vi "Starting.vi"(4 "Queue of Error":refnum<queue>, 6 "Queue of Self Attributes":refnum<queue>, 7 "Actor in":refnum<class "Actor.lvclass">, 10 "Attributes":refnum<class "Attributes.lvclass">) -> (0 "Error out":errorcluster, 5 "Actor out":refnum<class "Actor.lvclass">)   [LabVIEW 2025, in "jettl.lvlib" / "Transport.lvlib" / "Event.lvlib"]
uses:
  Event.lvlib
  Actor/Actor.lvclass
  Attributes/Attributes/Attributes.lvclass
  jettl.lvlib
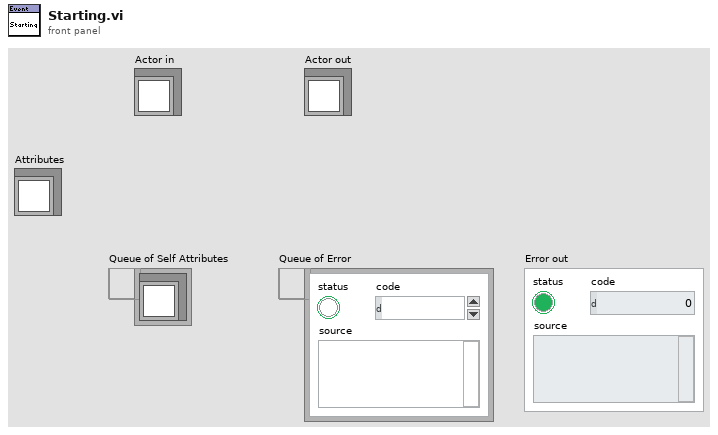
[diagram p1: front panel]
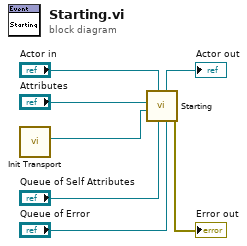
[diagram p0: block diagram]
diagram:
  n1 = call "Init Transport.vi"() -> ("Transport"=w1:refnum<class "Transport.lvclass">)  [unwired: 11 in]
  n2 = call "Starting.vi"("Queue of Error"="Queue of Error", "Queue of Self Attributes"="Queue of Self Attributes", "Actor in"="Actor in", "Transport"=w1, "Attributes"="Attributes") -> ("Error out"=→"Error out":errorcluster, "Actor out"=→"Actor out":refnum<class "Actor.lvclass">)  [unwired: 5 in]
